vi "Position Title String.vi"(8 "error in (no error)":errorcluster, 11 "String Ref":refnum<vi>) -> (0 "error out":errorcluster)   [LabVIEW 2014]
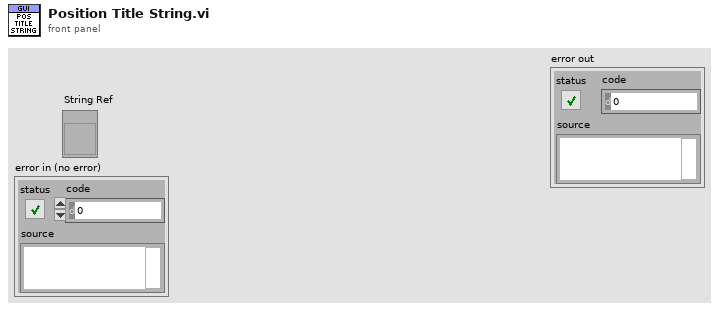
[diagram p1: front panel]
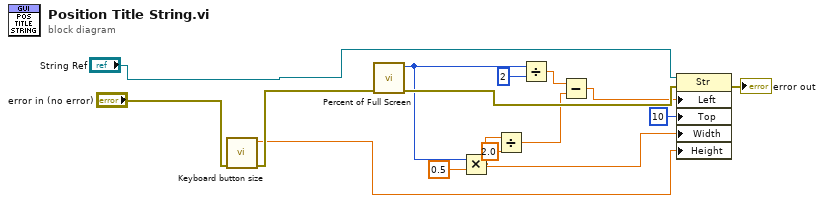
[diagram p0: block diagram]
diagram:
  n1 = call "Keyboard button size.vi"("error in (no error)"="error in (no error)") -> ("error out"=w2:errorcluster, "Key Height"=w1:dbl)  [unwired: 7 in, 2 out]
  n2 = call "Percent of Full Screen.vi"("error in (no error)"=w2) -> ("error out"=w13:errorcluster, "Right"=w9:i16)  [unwired: 8 in, 1 out]
  n3 = Multiply(x=w9, y=0.5) -> (x*y=w6:dbl)
  n4 = Divide(x=w6, y=2.0) -> (x/y=w4:dbl)
  n5 = Divide(x=w9, y=i16 2) -> (x/y=w14:dbl)
  n6 = Subtract(x=w14, y=w4) -> (x-y=w12:dbl)
  n7 = property class="Str"(reference="String Ref", error in=w13, "Left"=w12, "Top"=10 ("Position:Top"), "Width"=w6, "Height"=w1) -> (error out=→"error out":errorcluster)  [unwired: 1 out]
